vi "Channel Estimation.vi"(0 "subcarrier channels":T1, 2 "field map":T3, 4 "subcarrier timing":T2={"subcarrier index"=0, "OFDM symbol index"=0, "frequency offset index"=0.0, "OFDM symbol start"=TRUE, "valid"=TRUE}, 6 "bandwidth":enum16{"20MHz", "40MHz", "80MHz"}(ring), 10 "subcarrier index in":fxp<+/-,9,9>) -> (20 "subcarrier index":u8, 23 "channel estimate":T1, 24 "output valid":bool=TRUE, 26 "subcarrier index":fxp<+/-,9,9>)   [LabVIEW 2020]
panel:
  out "Imag":fxp<+/-,25,4>
  out "Real":fxp<+/-,25,4>
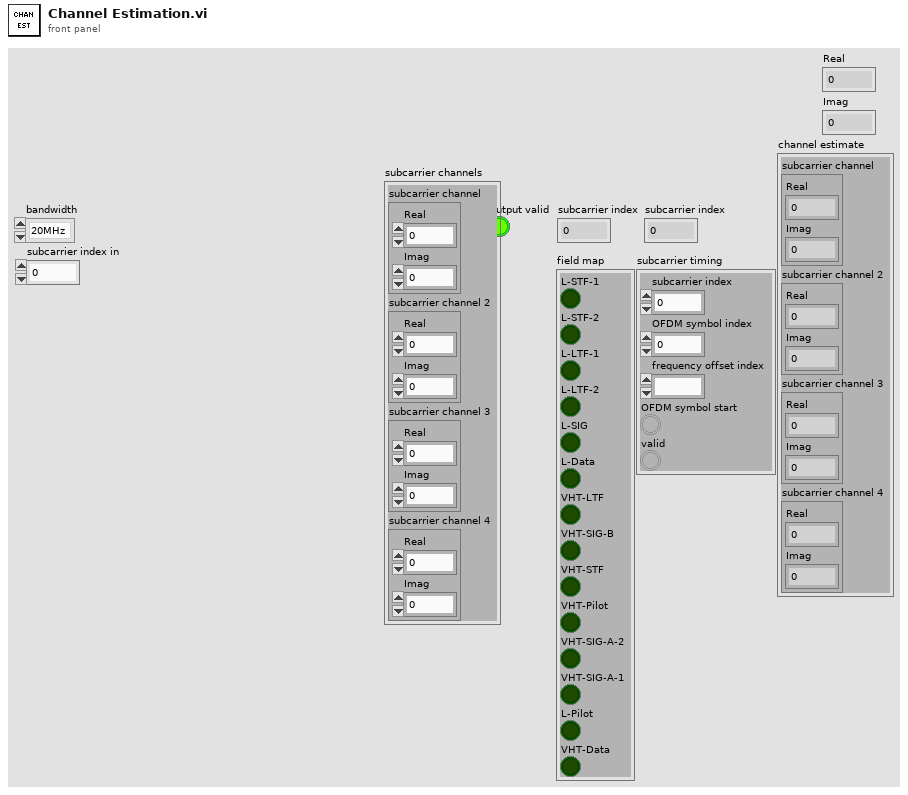
[diagram p1: front panel]
types:
  T1 = cluster{"subcarrier channel":cluster{"Real":fxp<+/-,25,4>, "Imag":fxp<+/-,25,4>}, "subcarrier channel 2":cluster{"Real":fxp<+/-,25,4>, "Imag":fxp<+/-,25,4>}, "subcarrier channel 3":cluster{"Real":fxp<+/-,25,4>, "Imag":fxp<+/-,25,4>}, "subcarrier channel 4":cluster{"Real":fxp<+/-,25,4>, "Imag":fxp<+/-,25,4>}}
  T2 = cluster{"subcarrier index":u8, "OFDM symbol index":u16, "frequency offset index":fxp<+/-,9,9>, "OFDM symbol start":bool, "valid":bool}
  T3 = cluster{"L-STF-1":bool, "L-STF-2":bool, "L-LTF-1":bool, "L-LTF-2":bool, "L-SIG":bool, "L-Data":bool, "VHT-LTF":bool, "VHT-SIG-B":bool, "VHT-STF":bool, "VHT-Pilot":bool, "VHT-SIG-A-2":bool, "VHT-SIG-A-1":bool, "L-Pilot":bool, "VHT-Data":bool}
  T4 = cluster{"BPSK constellation":bool, "not in list":bool}
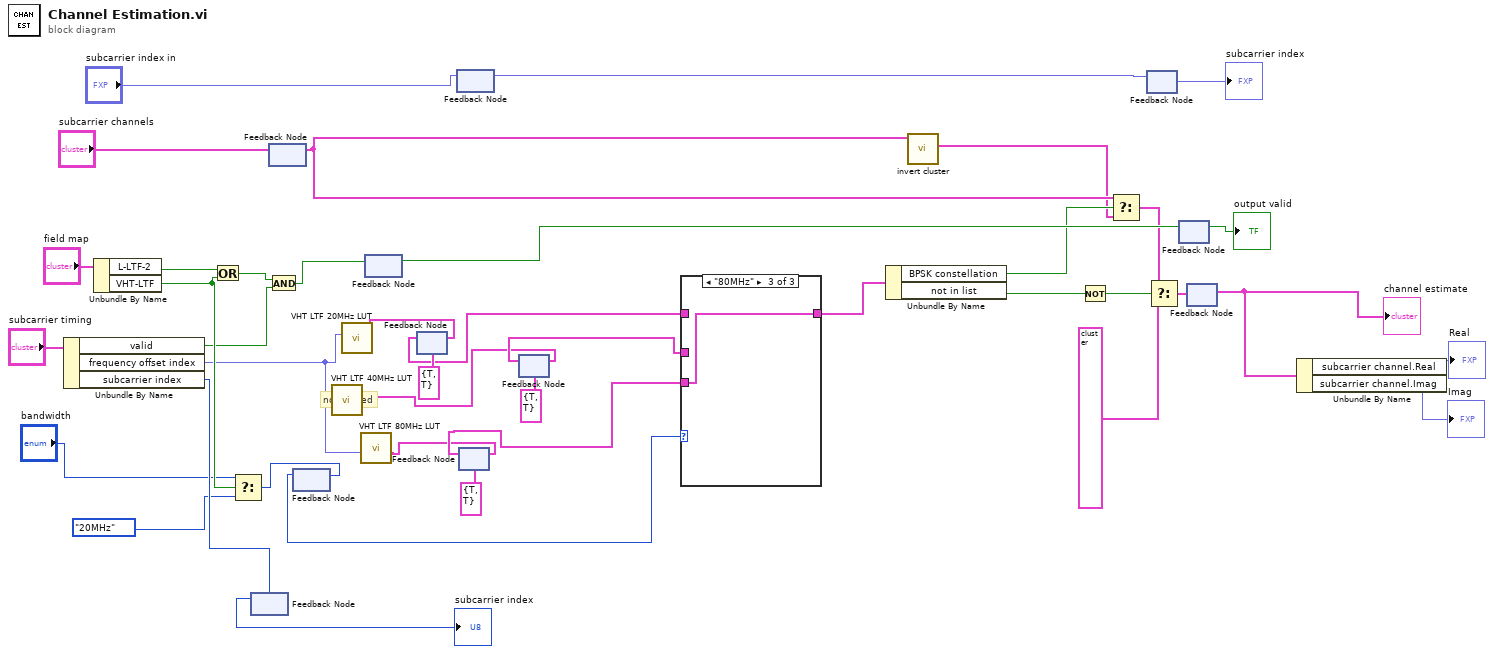
[diagram p0: block diagram]
diagram:
  # "not tested"
  n1 = Unbundle By Name("subcarrier timing") -> ("valid"=w35:bool, "frequency offset index"=w20:fxp<+/-,9,9>, "subcarrier index"=w33:u8)
  n2 = Unbundle By Name("field map") -> ("L-LTF-2"=w40:bool, "VHT-LTF"=w39:bool)
  n3 = Or(x=w40, y=w39) -> (x .or. y?=w36:bool)
  n4 = Select(t="bandwidth", s=w39, f=enum16{"20MHz", "40MHz", "80MHz"}."20MHz" ("bandwidth")) -> (s? t:f=w38:enum16{"20MHz", "40MHz", "80MHz"})
  n5 = feedback #1() -> (→"subcarrier index":u8)  [unwired: 1 in]
  n6 = feedback-in #1(w33) -> ()
  n7 = feedback #2() -> (w3:T1)  [unwired: 1 in]
  n8 = feedback-in #2("subcarrier channels") -> ()
  n9 = And(x=w36, y=w35) -> (x .and. y?=w34:bool)
  n10 = feedback #3() -> (w27:enum16{"20MHz", "40MHz", "80MHz"})  [unwired: 1 in]
  n11 = feedback-in #3(w38) -> ()
  n12 = call "VHT LTF 40MHz LUT.vi"("frequency offset index"=w20) -> ("VHT LTF symbol"=w21:T4)  [unwired: 10 in]
  n13 = call "VHT LTF 20MHz LUT.vi"("frequency offset index"=w20) -> ("VHT LTF symbol"=w30:T4)  [unwired: 10 in]
  n14 = call "VHT LTF 80MHz LUT.vi"("frequency offset index"=w20) -> ("VHT LTF symbol"=w19:T4)  [unwired: 10 in]
  n15 = feedback #4() -> (w17:bool)  [unwired: 1 in]
  n16 = feedback-in #4(w34) -> ()
  n17 = feedback #5(T4 {"BPSK constellation"=TRUE, "not in list"=TRUE} ("Data")) -> (w26:T4)
  n18 = feedback-in #5(w30) -> ()
  n19 = feedback #6() -> (w8:fxp<+/-,9,9>)  [unwired: 1 in]
  n20 = feedback-in #6("subcarrier index in") -> ()
  n21 = feedback #7(T4 {"BPSK constellation"=TRUE, "not in list"=TRUE} ("Data")) -> (w22:T4)
  n22 = feedback-in #7(w19) -> ()
  n23 = feedback #8(T4 {"BPSK constellation"=TRUE, "not in list"=TRUE} ("Data")) -> (w24:T4)
  n24 = feedback-in #8(w21) -> ()
  n25 = case shown="\"80MHz\"" w27 {
    tunnel: w26 -> [w42 _ _]
    tunnel: w24 -> [_ w43 _]
    tunnel: w22 -> [_ _ w44]
    tunnel: [w42 w43 w44] -> w10
    frame "20MHz", Default {
    }
    frame "40MHz" {
    }
    frame "80MHz" {
    }
  }
  n26 = Unbundle By Name(w10) -> ("BPSK constellation"=w15:bool, "not in list"=w14:bool)
  n27 = call "invert cluster.vi"("subcarrier channels"=w3) -> ("subcarrier channels out"=w2:T1)  [unwired: 10 in]
  n28 = Not(x=w14) -> (.not. x?=w13:bool)
  n29 = Select(t=w3, s=w15, f=w2) -> (s? t:f=w12:T1)
  n30 = feedback #9() -> (→"subcarrier index":fxp<+/-,9,9>)  [unwired: 1 in]
  n31 = feedback-in #9(w8) -> ()
  n32 = Select(t=w12, s=w13, f=T1 {"subcarrier channel"={"Real"=0.0, "Imag"=0.0}, "subcarrier channel 2"={"Real"=0.0, "Imag"=0.0}, "subcarrier channel 3"={"Real"=0.0, "Imag"=0.0}, "subcarrier channel 4"={"Real"=0.0, "Imag"=0.0}}) -> (s? t:f=w11:T1)
  n33 = feedback #10() -> (→"output valid":bool)  [unwired: 1 in]
  n34 = feedback-in #10(w17) -> ()
  n35 = feedback #11() -> (w7:T1)  [unwired: 1 in]
  "channel estimate" <- w7
  n36 = feedback-in #11(w11) -> ()
  n37 = Unbundle By Name(w7) -> ("subcarrier channel.Real"=→"Real":fxp<+/-,25,4>, "subcarrier channel.Imag"=→"Imag":fxp<+/-,25,4>)
